vi "Main.vi"() -> ()   [LabVIEW 2020]
uses:
  <vilib>/userdefined/High Color/IMAQdx.ctl
  <vilib>/vision/driver/NI_Vision_Acquisition_Software.lvlib
  <vilib>/vision/NI_Vision_Development_Module.lvlib
panel:
  out "错误输出":errorcluster
  in  "停止":bool
  out "Image":T1(plugin-control)
  out "Read String":string
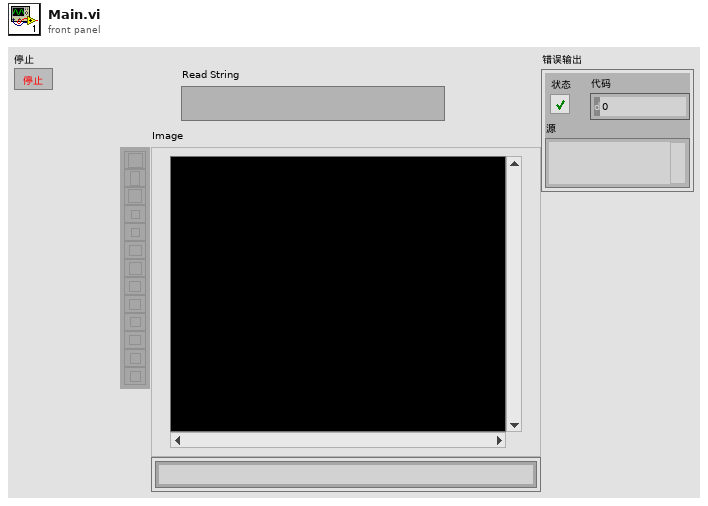
[diagram p1: front panel]
types:
  T1 = typedef "IMAQ Image.ctl" = refnum<image>
  T2 = typedef "IMAQ Rectangle" = cluster{"Left":i32, "Top":i32, "Right":i32, "Bottom":i32, "Rotation":dbl}
  T3 = typedef "IMAQdx.ctl" = refnum<k21>
  T4 = typedef "IMAQ OCR Session.ctl" = refnum<k1>
  T5 = typedef "ROI Descriptor" = cluster{"Global Rectangle":i32[], "Contours":cluster{"ID":enum32{"External", "Internal"}, "Type":u32, "Coordinates":i32[]}[]}
  T6 = cluster{"Global Rectangle":i32[], "Contours":cluster{"ID":enum32{"External", "Internal"}, "Type":u32, "Coordinates":i32[]}[]}
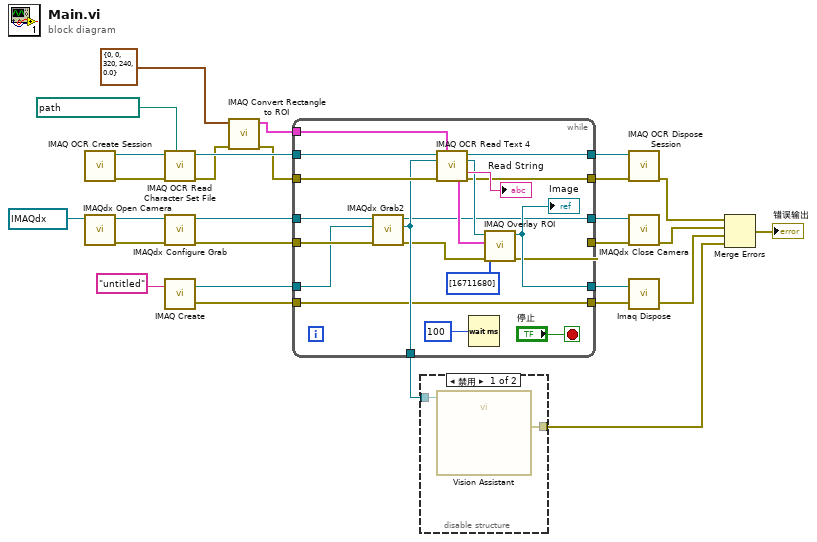
[diagram p0: block diagram]
diagram:
  n1 = call "IMAQ OCR Create Session"() -> ("error out"=w23:errorcluster, "IMAQ OCR Session"=w24:T4)  [unwired: 10 in]
  n2 = call <vilib>:"IMAQdx Open Camera.vi"("Session In"=T3 "cam1") -> ("error out"=w25:errorcluster, "Session Out"=w26:T3)  [unwired: 9 in]
  n3 = call "IMAQ OCR Read Character Set File"("File Path"=path "E:/朱晨辉/个人资料/01-计算机编程/00-上位机开发/02-基础知识/09-基于VISION的图像采集V2020/09-车牌字母识别/Hardware/字母识别.abc", "error in (no error)"=w23, "IMAQ OCR Session"=w24) -> ("error out"=w16:errorcluster, "IMAQ OCR Session (dup)"=w17:T4)  [unwired: 6 in, 1 out]
  n4 = call <vilib>:"IMAQdx Configure Grab.vi"("error in"=w25, "Session In"=w26) -> ("error out"=w19:errorcluster, "Session Out"=w20:T3)  [unwired: 8 in]
  n5 = call "IMAQ Create"("Image Name"="untitled") -> ("New Image"=w18:T1, "error out"=w12:errorcluster)  [unwired: 4 in]
  n6 = call "IMAQ Convert Rectangle to ROI"("error in (no error)"=w16, "Rectangle"=T2 {"Left"=0, "Top"=0, "Right"=320, "Bottom"=240, "Rotation"=0.0}) -> ("error out"=w15:errorcluster, "ROI Descriptor"=w14:T5)  [unwired: 7 in]
  n7 = while {
    tunnel: w20 -> [w48]
    tunnel: w19 -> [w47]
    tunnel: w18 -> [w46]
    tunnel: w17 -> [w45]
    tunnel: w15 -> [w44]
    tunnel: w14 -> [w43]
    tunnel: [w42] -> w13
    tunnel: w12 -> [w36]
    tunnel: [w36] -> w11
    tunnel: [w35] -> w10
    tunnel: [w34] -> w9
    tunnel: [w33] -> w8
    tunnel: [w31] -> w7
    tunnel: [w30] -> w6
    stop <- "停止" stop-if-true
    n8 = call <vilib>:"IMAQdx Grab2.vi"("error in"=w47, "Image In"=w46, "Session In"=w48) -> ("error out"=w32:errorcluster, "Image Out"=w42:T1, "Session Out"=w30:T3)  [unwired: 5 in, 1 out]
    n9 = call "IMAQ OCR Read Text 4"("IMAQ OCR Session"=w45, "ROI Descriptor"=w43, "Image"=w42, "error in (no error)"=w44) -> ("IMAQ OCR Session (dup)"=w34:T4, "Image (dup)"=w40:T1, "Read String"=→"Read String":string, "ROI Bounding Characters"=w39:T6, "error out"=w33:errorcluster)  [unwired: 5 in, 2 out]
    n10 = Wait (ms)(milliseconds to wait=u32 100 ("等待时间（毫秒）")) -> ()  [unwired: 1 out]
    n11 = call "IMAQ Overlay ROI"("Colors (Green)"=u32[] [16711680], "error in (no error)"=w32, "ROI Descriptor"=w39, "Image"=w40) -> ("error out"=w31:errorcluster, "Image Out"=w35:T1)  [unwired: 6 in]
    "Image" <- w35
  }
  n12 = disable-structure shown="禁用" {
    disable-tunnel: w13 -> [w50 _]
    disable-tunnel: [w49 _] -> w2
    frame Disabled {
      n13 = call "Vision Assistant"("Image In"=w50) -> ("error out"=w49:errorcluster)  [unwired: 25 in, 1 out]
    }
    frame Enabled {
    }
  }
  n14 = call "IMAQ OCR Dispose Session"("error in (no error)"=w8, "IMAQ OCR Session"=w9) -> ("error out"=w5:errorcluster)  [unwired: 9 in]
  n15 = call <vilib>:"IMAQdx Close Camera.vi"("error in"=w7, "Session In"=w6) -> ("error out"=w4:errorcluster)  [unwired: 9 in]
  n16 = call "Imaq Dispose"("Image"=w10, "error in (no error)"=w11) -> ("error out"=w3:errorcluster)  [unwired: 4 in]
  n17 = Merge Errors(w5, w4, w3, w2) -> (→"错误输出":errorcluster)
